vi "continou_sampling_diag (1).vi"(6 "samples per channel":i32=1000, 7 "rate":dbl=1000.0 format="%0.2f", 8 "error in":errorcluster, 11 "task/channels in":refnum<k21>) -> (0 "error out":errorcluster, 2 "data":dbl[][](array[numeric]) format="%0.2f", 3 "task out":refnum<k21>)   [LabVIEW 2011]
uses:
  <vilib>/DAQmx/read.llb/DAQmx Read (Analog 2D DBL NChan NSamp).vi
  <vilib>/DAQmx/configure/timing.llb/DAQmx Timing (Sample Clock).vi
  <vilib>/DAQmx/miscellaneous.llb/DAQmx Fill In Error Info.vi
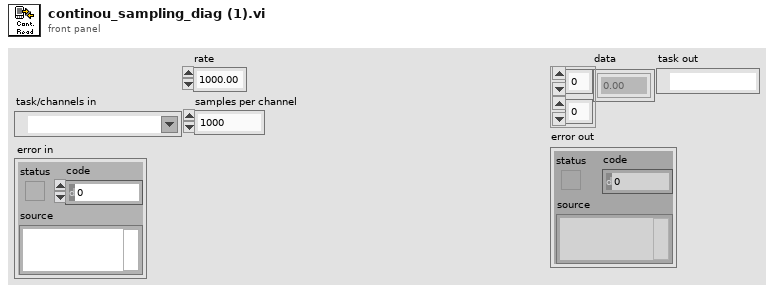
[diagram p1: front panel]
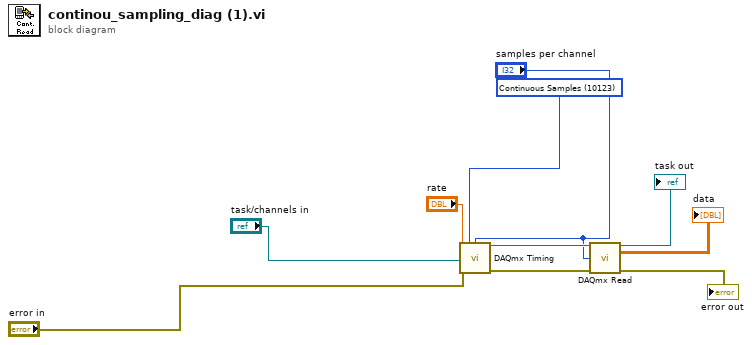
[diagram p0: block diagram]
diagram:
  w9 = 10123 items=["Finite Samples"=10178, "Continuous Samples"=10123, "Hardware Timed Single Point"=12522] ("sample mode")
  n1 = call-poly <vilib>:"DAQmx Timing.vi"("task/channels in"="task/channels in", "sample mode"=w9, "samples per channel"="samples per channel", "rate"="rate", "error in"="error in") -> ("task out"=w8:refnum<k21>, "error out"=w7:errorcluster)  [unwired: 9 in]
  n2 = call-poly <vilib>:"DAQmx Read.vi"("task/channels in"=w8, "number of samples per channel"="samples per channel", "error in"=w7) -> ("task out"=→"task out":refnum<k21>, "data"=→"data":dbl[][], "error out"=→"error out":errorcluster)  [unwired: 10 in]
